vi "16TVTI-WriteSetpoint.vi"(2 "Set point":dbl[unit] min=0.0 format="%.2f", 3 "Instrument address":T1) -> (0 "Instrument address (out)":T1)   [LabVIEW 2016]
doc: "Sets the setpoint for the specified channel of the ITC."
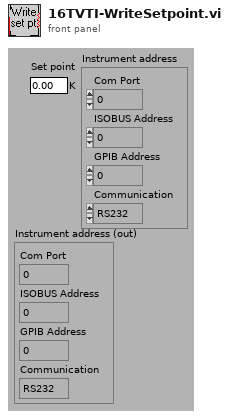
[diagram p1: front panel]
types:
  T1 = cluster{"Com Port":i32, "ISOBUS Address":i32, "GPIB Address":i16, "Communication":enum16{"RS232", "ISOBUS", "GPIB", "Gateway"}}
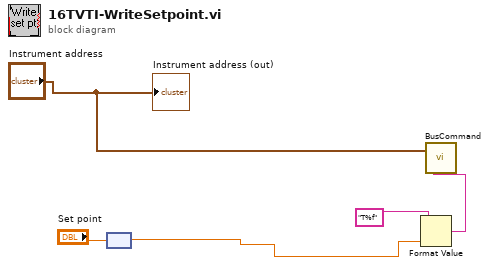
[diagram p0: block diagram]
diagram:
  n1 = node("Set point") -> (w5:dbl)
  n2 = Format Value(format string="T%f", value (0)=w5) -> (output string=w2:string)  [unwired: 1 in]
  n3 = call "BusCommand.vi"("Command"=w2, "Instrument address (in)"="Instrument address") -> ()  [unwired: 2 out]
  "Instrument address (out)" <- "Instrument address"
